vi "Sensor Case Selector.vi"(2 "Avoid Distance":dbl=0.5 format="%#_13g", 3 "FR":dbl format="%#_13g", 4 "FL":dbl format="%#_13g") -> (0 "Case":u8, 1 "Obstacle Detected":bool)   [LabVIEW 2013]
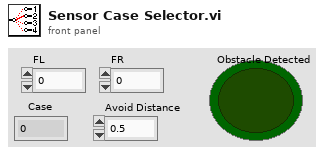
[diagram p1: front panel]
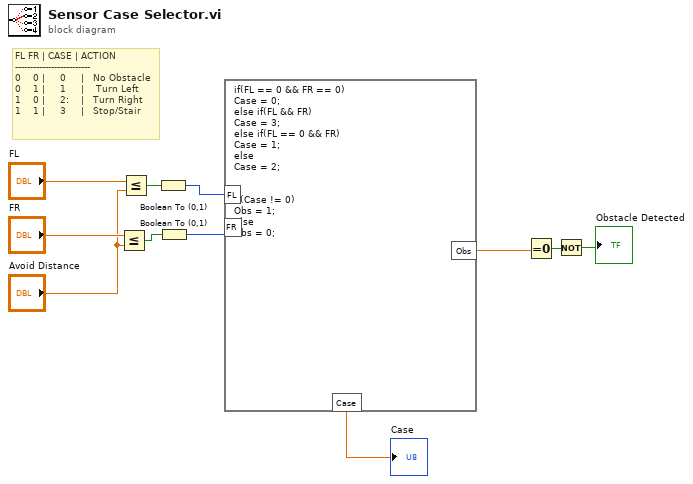
[diagram p0: block diagram]
diagram:
  # "FL FR | CASE | ACTION\n-------------------------\n0    0 |     0     |   No Obstacle\n0    1 |     1     |    Turn Left\n1    0 |     2:    |   Turn Right\n1    1 |     3     |   Stop/Stair"
  n1 = Less Or Equal?(x="FR", y="Avoid Distance") -> (x <= y?=w4:bool)
  n2 = Less Or Equal?(x="FL", y="Avoid Distance") -> (x <= y?=w5:bool)
  n3 = Boolean To (0,1)(Boolean=w5) -> (0, 1=w11:i16)
  n4 = Boolean To (0,1)(Boolean=w4) -> (0, 1=w10:i16)
  n5 = formula code="if(FL == 0 && FR == 0)\nCase = 0;\nelse if(FL && FR)\nCase = 3;\nelse if(FL == 0 && FR)\nCase = 1;\nelse\nCase = 2;\n\n\nif(Case != 0)\nObs = 1;\nelse\nObs = 0;"("FL"=w11, "FR"=w10) -> ("Case"=→"Case":dbl, "Obs"=w3:dbl)
  n6 = Equal To 0?(x=w3) -> (x = 0?=w2:bool)
  n7 = Not(x=w2) -> (.not. x?=→"Obstacle Detected":bool)
